vi "Smooth Background WFRM DBL.vi"(8 "Error In":errorcluster, 9 "HP F":dbl format="%#_6p", 10 "LP  F":dbl=0.001 format="%#_6p", 11 "Data":waveform(dbl)) -> (0 "Error Out":errorcluster, 3 "Data out":waveform(dbl))   [LabVIEW 2016]
uses:
  <vilib>/Analysis/3filter.llb/Filter Structure Type.ctl
  <vilib>/measure/macond.llb/IIR Filter for 1 Chan.vi
  <vilib>/measure/NI_MAPro.lvlib
  <vilib>/Analysis/NI_AALBase.lvlib
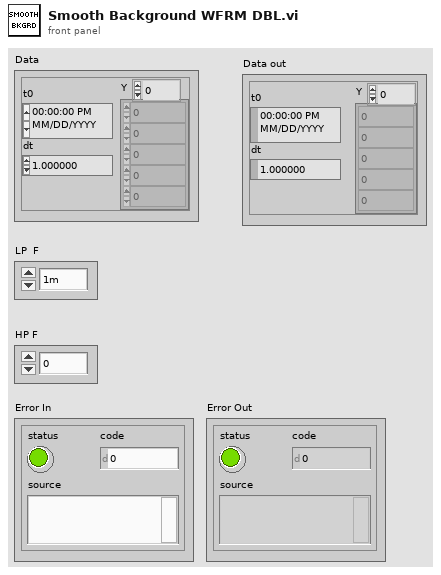
[diagram p1: front panel]
types:
  T1 = typedef "NI_AALBase.lvlib/Filter Structure Type.ctl" = u16
  T2 = cluster{"Topology":enum16{"Off", "Butterworth", "Chebyshev", "Inverse Chebyshev", "Elliptic", "Bessel"}, "Type":enum16{"Lowpass", "Highpass", "Bandpass", "Bandstop"}, "Order":i32, "Lower Fc":dbl, "Upper Fc":dbl, "PB Ripple":dbl, "SB Attenuation":dbl}
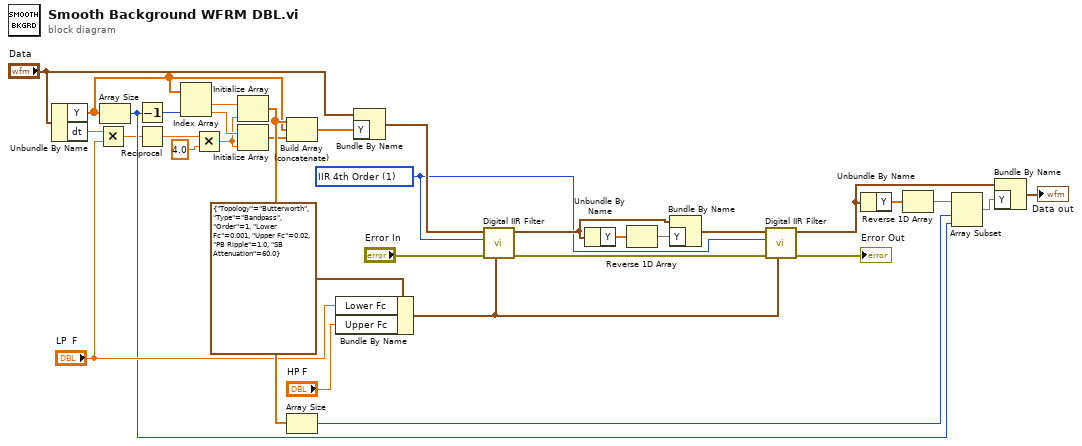
[diagram p0: block diagram]
diagram:
  w19 = T1 1 items=["IIR 2nd Order"=0, "IIR 4th Order"=1, "Auto Select"=10] ("filter structure option")
  n1 = Unbundle By Name("Data") -> ("Y"=w7:dbl[], "dt"=w4:dbl)
  n2 = Multiply(x=w4, y="LP  F") -> (x*y=w5:dbl)
  n3 = Array Size(array=w7) -> (size(s)=w14:i32)
  n4 = Decrement(x=w14) -> (x-1=w13:i32)
  n5 = Reciprocal(x=w5) -> (1/x=w29:dbl)
  n6 = Index Array(array=w7, index #2=w13) -> (element #1=w31:dbl, element #2=w12:dbl)  [unwired: 1 in]
  n7 = Multiply(x=w29, y=4.0) -> (x*y=w11:dbl)
  n8 = Initialize Array(w31, w11) -> (w33:dbl[])
  n9 = Initialize Array(w12, w11) -> (w10:dbl[])
  n10 = Build Array (concatenate)(w33, w7, w10) -> (w32:dbl[])
  n11 = Array Size(array=w33) -> (size(s)=w15:i32)
  n12 = Bundle By Name(cluster=T2 {"Topology"=enum."Butterworth", "Type"=enum."Bandpass", "Order"=1, "Lower Fc"=0.001, "Upper Fc"=0.02, "PB Ripple"=1.0, "SB Attenuation"=60.0} ("IIR filter specifications"), "Lower Fc"="LP  F", "Upper Fc"="HP F") -> (w20:T2)
  n13 = Bundle By Name(cluster="Data", "Y"=w32) -> (w28:waveform(dbl))
  n14 = call-poly <vilib>:"Digital IIR Filter.vi"("IIR filter specifications"=w20, "error in (no error)"="Error In", "filter structure option"=w19, "signal in"=w28) -> ("error out"=w18:errorcluster, "signal out"=w23:waveform(dbl))  [unwired: 5 in, 1 out]
  n15 = Unbundle By Name(w23) -> ("Y"=w24:dbl[])
  n16 = Reverse 1D Array(array=w24) -> (reversed array=w22:dbl[])
  n17 = Bundle By Name(cluster=w23, "Y"=w22) -> (w21:waveform(dbl))
  n18 = call-poly <vilib>:"Digital IIR Filter.vi"("IIR filter specifications"=w20, "error in (no error)"=w18, "filter structure option"=w19, "signal in"=w21) -> ("error out"=→"Error Out":errorcluster, "signal out"=w3:waveform(dbl))  [unwired: 5 in, 1 out]
  n19 = Unbundle By Name(w3) -> ("Y"=w17:dbl[])
  n20 = Reverse 1D Array(array=w17) -> (reversed array=w16:dbl[])
  n21 = Array Subset(array=w16, index=w15, length=w14) -> (w1:dbl[])
  n22 = Bundle By Name(cluster=w3, "Y"=w1) -> (→"Data out":waveform(dbl))
